vi "exercícios1.vi"() -> ()   [LabVIEW 2018]
panel:
  out "Waveform Chart":dbl(graph)
  out "Gráfico":cluster{"X":dbl, "Y":dbl}[](graph)
  in  "Fechar":bool
  in  "Chave":bool
  in  "Volume":i64(slide) scale=0.0..100.0
  out "Boolean":bool
  out "Gauge":i32(knob) scale=10.0..225.0
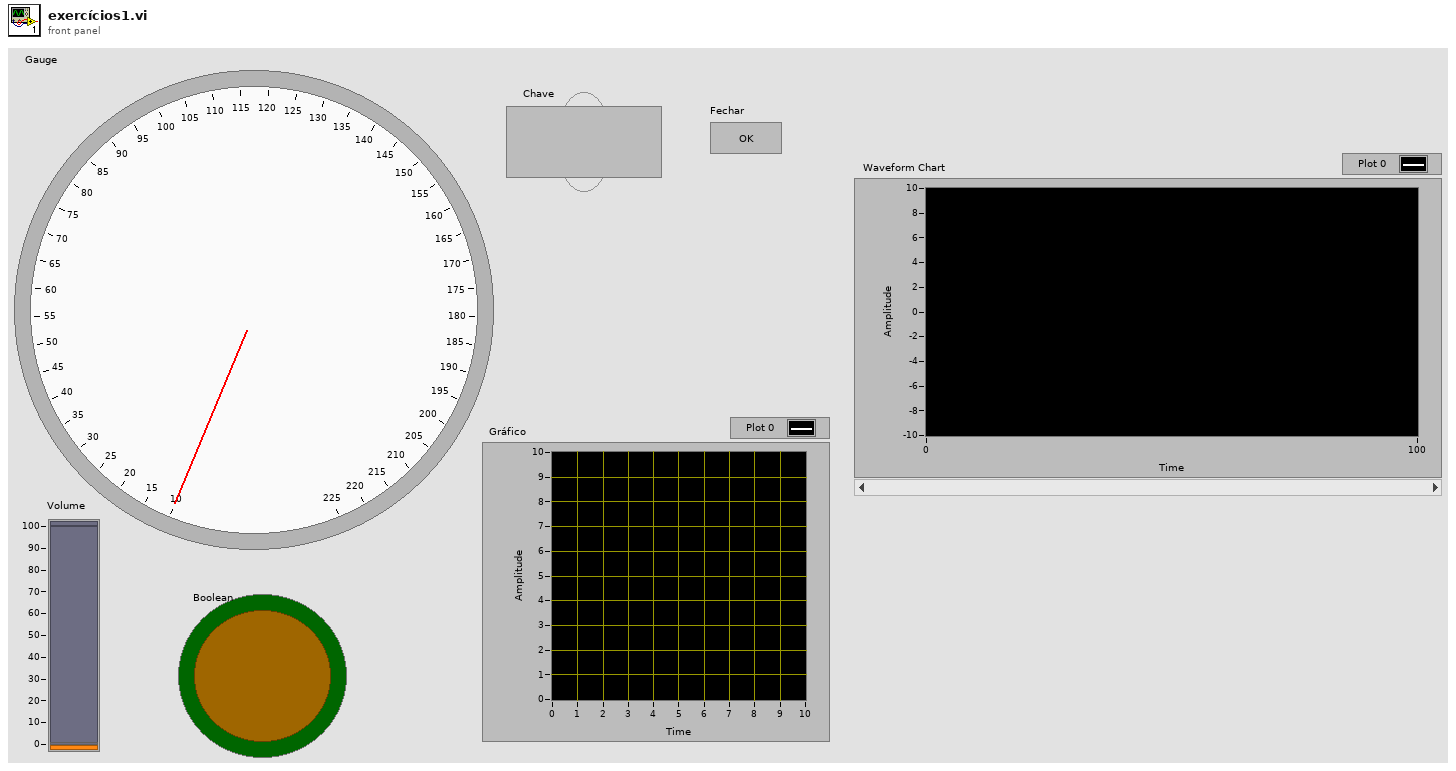
[diagram p1: front panel]
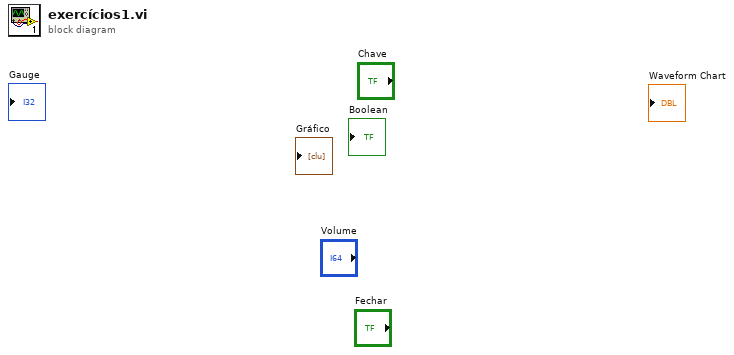
[diagram p0: block diagram]
diagram:
